vi "newTestStandStep.vi"(0 "Engine reference":refnum<k7>, 1 "adapterKeyNameVal":string, 5 "stepType":string="Action", 7 "Step Name":string, 9 "Requirement":string, 11 "error in":errorcluster, 12 "RecordResult":bool=TRUE, 13 "Record Req":bool=TRUE) -> (4 "Engine reference(out)":refnum<k7>, 6 "NewStep (out)":refnum<k7>, 15 "error out":errorcluster)   [LabVIEW 2011]
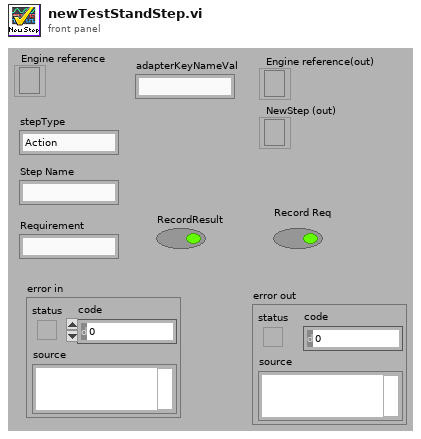
[diagram p1: front panel]
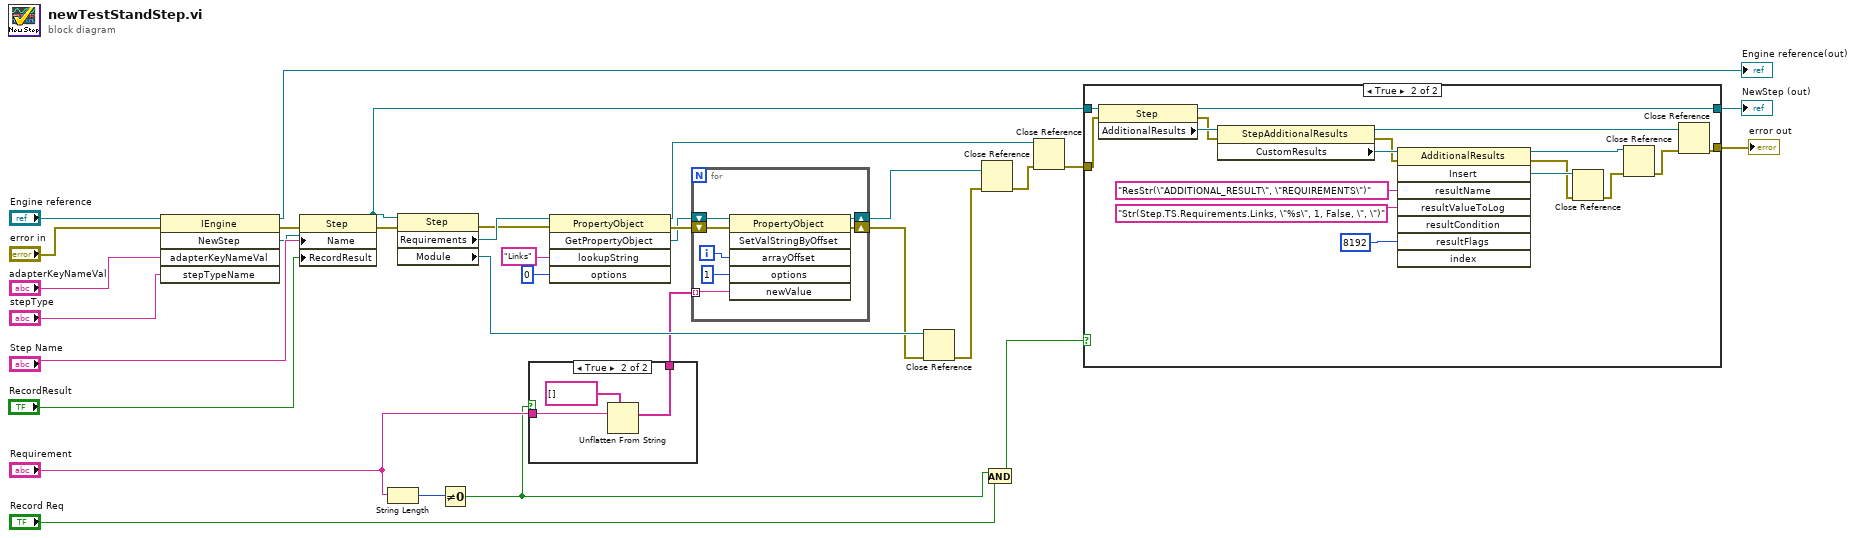
[diagram p0: block diagram]
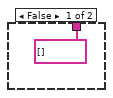
[diagram p2: hidden frame]
diagram:
  n1 = invoke class="IEngine" method="NewStep"(reference="Engine reference", error in="error in", "adapterKeyNameVal"="adapterKeyNameVal", "stepTypeName"="stepType") -> (reference out=→"Engine reference(out)":refnum<k7>, error out=w27:errorcluster, "NewStep"=w19:refnum<k7>)  [unwired: 1 in, 2 out]
  n2 = property class="Step"(reference=w19, error in=w27, "Name"="Step Name", "RecordResult"="RecordResult") -> (reference out=w10:refnum<k7>, error out=w17:errorcluster)
  n3 = String Length(string="Requirement") -> (length=w4:i32)
  n4 = property class="Step"(reference=w10, error in=w17) -> (error out=w16:errorcluster, "Requirements"=w18:refnum<k7>, "Module"=w15:refnum<k7>)  [unwired: 1 out]
  n5 = Not Equal To 0?(x=w4) -> (x != 0?=w1:bool)
  n6 = case shown="True" w1 {
    tunnel: "Requirement" -> [_ w36]
    tunnel: [string[] [] w35] -> w2
    frame False {
    }
    frame True {
      n7 = Unflatten From String(type=string[] [], binary string=w36) -> (value=w35:string[])  [unwired: 3 in, 2 out]
    }
  }
  n8 = invoke class="PropertyObject" method="GetPropertyObject"(reference=w18, error in=w16, "lookupString"="Links", "options"=0) -> (reference out=w22:refnum<k7>, error out=w32:errorcluster, "GetPropertyObject"=w31:refnum<k7>)  [unwired: 1 in, 2 out]
  n9 = for {
    tunnel: w2 -> [w38] mode=indexing
    shift-right: [w40] -> w23
    shift-left: w31 -> [w41]
    shift-right: [w39] -> w13
    shift-left: w32 -> [w43]
    i -> [w37]
    n10 = invoke class="PropertyObject" method="SetValStringByOffset"(reference=w41, error in=w43, "arrayOffset"=w37, "options"=1, "newValue"=w38) -> (reference out=w40:refnum<k7>, error out=w39:errorcluster)  [unwired: 1 in, 4 out]
  }
  n11 = Close Reference(reference=w15, error in (no error)=w13) -> (error out=w14:errorcluster)
  n12 = Close Reference(reference=w23, error in (no error)=w14) -> (error out=w21:errorcluster)
  n13 = And(x=w1, y="Record Req") -> (x .and. y?=w3:bool)
  n14 = Close Reference(reference=w22, error in (no error)=w21) -> (error out=w8:errorcluster)
  n15 = case shown="True" w3 {
    tunnel: w10 -> [w45 w50]
    tunnel: [w45 w49] -> w9
    tunnel: w8 -> [w44 w48]
    tunnel: [w44 w47] -> w7
    frame False {
    }
    frame True {
      n16 = property class="Step"(reference=w50, error in=w48) -> (reference out=w49:refnum<k7>, error out=w46:errorcluster, "AdditionalResults"=w62:refnum<k7>)
      n17 = property class="StepAdditionalResults"(reference=w62, error in=w46) -> (reference out=w54:refnum<k7>, error out=w60:errorcluster, "CustomResults"=w61:refnum<k7>)
      n18 = invoke class="AdditionalResults" method="Insert"(reference=w61, error in=w60, "resultName"="ResStr(\"ADDITIONAL_RESULT\", \"REQUIREMENTS\")", "resultValueToLog"="Str(Step.TS.Requirements.Links, \"%s\", 1, False, \", \")", "resultFlags"=8192) -> (reference out=w56:refnum<k7>, error out=w58:errorcluster, "Insert"=w59:refnum<k7>)  [unwired: 3 in, 5 out]
      n19 = Close Reference(reference=w59, error in (no error)=w58) -> (error out=w57:errorcluster)
      n20 = Close Reference(reference=w56, error in (no error)=w57) -> (error out=w55:errorcluster)
      n21 = Close Reference(reference=w54, error in (no error)=w55) -> (error out=w47:errorcluster)
    }
  }
  "error out" <- w7
  "NewStep (out)" <- w9
